vi "EXTRACT-DATA-UINT16.vi"(2 "UINT16":u16, 7 "Data":u8[](array[numeric])) -> (4 "Value":u16, 8 "Min":u16, 10 "Max":u16, 15 "Inc":u16)   [LabVIEW 2019]
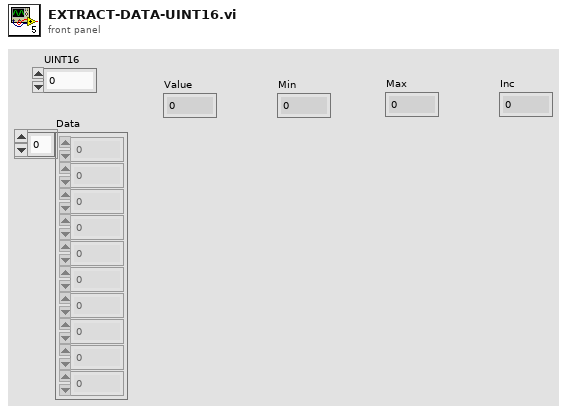
[diagram p1: front panel]
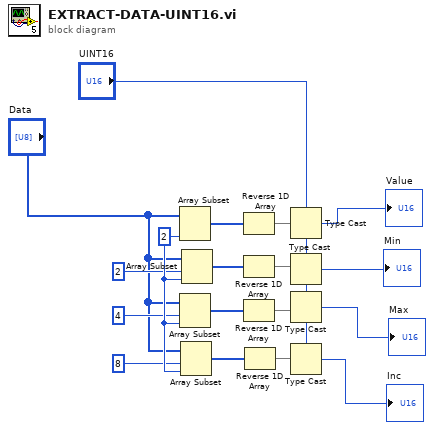
[diagram p0: block diagram]
diagram:
  w9 = 2 ("length")
  n1 = Array Subset(array="Data", length=w9) -> (w5:u8[])  [unwired: 1 in]
  n2 = Array Subset(array="Data", index=4, length=w9) -> (w4:u8[])
  n3 = Array Subset(array="Data", index=8, length=w9) -> (w10:u8[])
  n4 = Array Subset(array="Data", index=2, length=w9) -> (w3:u8[])
  n5 = Reverse 1D Array(array=w5) -> (reversed array=w11:u8[])
  n6 = Reverse 1D Array(array=w3) -> (reversed array=w12:u8[])
  n7 = Reverse 1D Array(array=w4) -> (reversed array=w13:u8[])
  n8 = Reverse 1D Array(array=w10) -> (reversed array=w14:u8[])
  n9 = Type Cast(type="UINT16", x=w11) -> (*(type *) &x=→"Value":u16)
  n10 = Type Cast(type="UINT16", x=w12) -> (*(type *) &x=→"Min":u16)
  n11 = Type Cast(type="UINT16", x=w13) -> (*(type *) &x=→"Max":u16)
  n12 = Type Cast(type="UINT16", x=w14) -> (*(type *) &x=→"Inc":u16)
